vi "H036 Harsh Pandit SCADA Lab 2a Sem 6.vi"() -> ()   [LabVIEW 2018]
panel:
  out "EXNOR":bool
  out "EXOR":bool
  out "NOR":bool
  out "NAND":bool
  in  "B":bool
  in  "A":bool
  # "Experiment 2a: Develope a HMI to perform logical operations like NAND, NOR, EXOR and EXNOR operations"
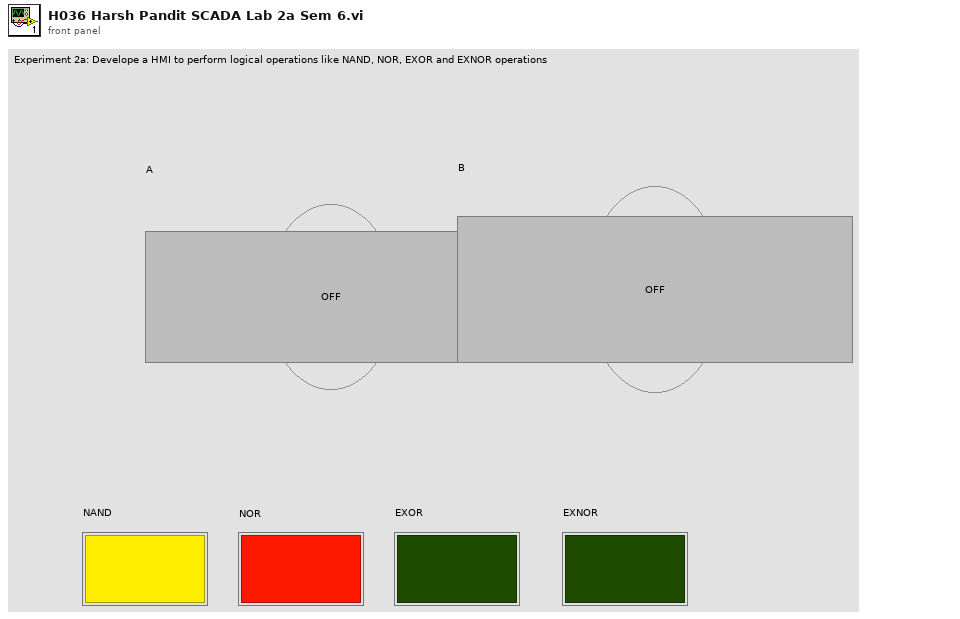
[diagram p1: front panel]
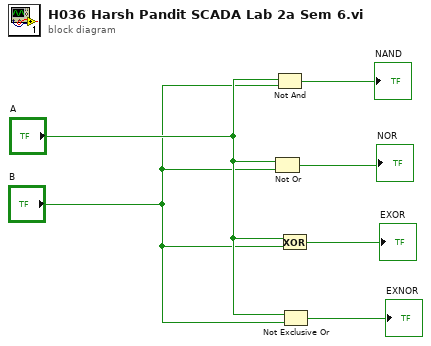
[diagram p0: block diagram]
diagram:
  n1 = Not Or(1:"B", 2:"A") -> (0:→"NOR":bool)
  n2 = Not And(1:"B", 2:"A") -> (0:→"NAND":bool)
  n3 = Exclusive Or(1:"B", 2:"A") -> (0:→"EXOR":bool)
  n4 = Not Exclusive Or(1:"B", 2:"A") -> (0:→"EXNOR":bool)
